vi "Get VS Amplitude String.vi"(8 "error in (no error)":errorcluster, 10 "text":string, 11 "index":i32) -> (0 "error out":errorcluster, 2 "text out":string, 3 "function return":u32)   [LabVIEW 2014, in "atmcd32d.lvlib"]
doc: "unsigned int WINAPI GetVSAmplitudeString(int index, char * text);"
uses:
  atmcd32d.lvlib
  atmcd32d.dll
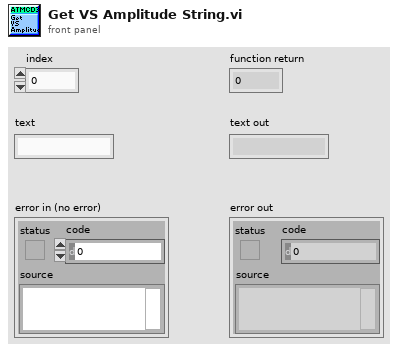
[diagram p1: front panel]
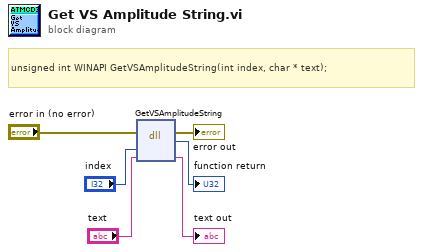
[diagram p0: block diagram]
diagram:
  # "unsigned int WINAPI GetVSAmplitudeString(int index, char * text);"
  n1 = dll-call lib="C:/Users/Bakir/Documents/Lambda2-Testing/lib/Andorlib/atmcd32d.*" fn="GetVSAmplitudeString"(error in="error in (no error)", "index"="index", "text"="text") -> (error out=→"error out":errorcluster, →"function return":u32, "text"=→"text out":string)  [unwired: 3 in, 1 out]
